vi "Test Run 1.vi"() -> ()   [LabVIEW 2009]
panel:
  out "Program Counter":u16 format="%x"
  out "Device Vcc":i32
  out "error out 2":errorcluster
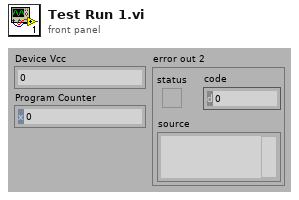
[diagram p1: front panel]
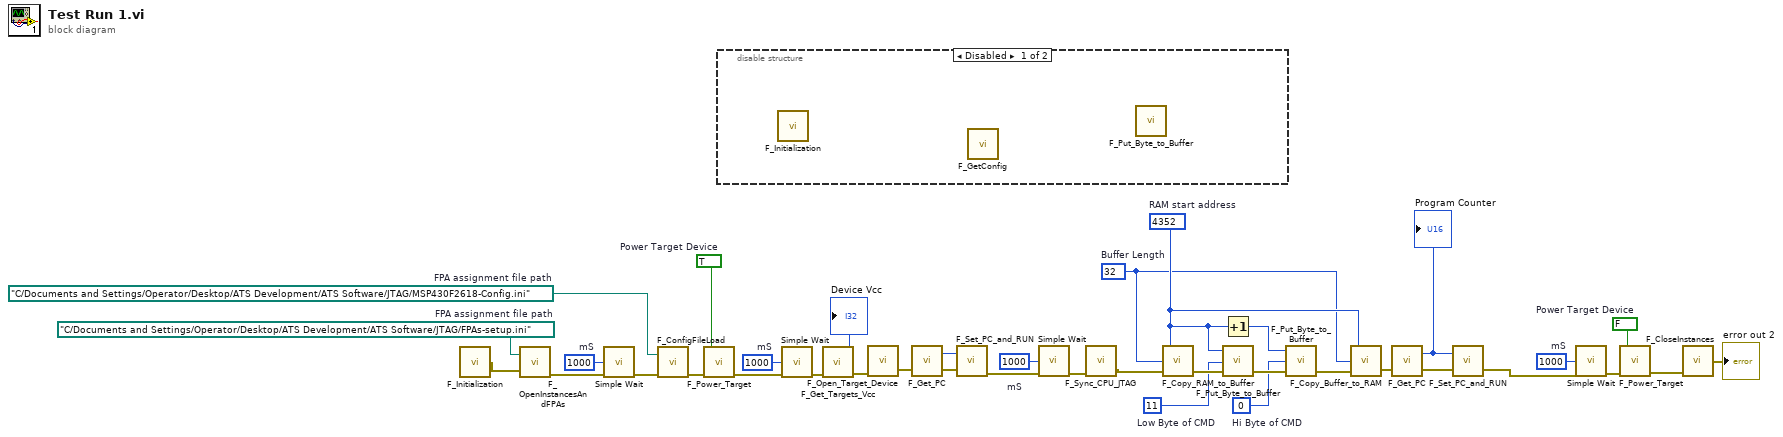
[diagram p0: block diagram]
diagram:
  w6 = u32 1000  # mS
  w15 = u32 1000  # mS
  w19 = u16 0  # Hi Byte of CMD
  w20 = u16 11  # Low Byte of CMD
  w16 = u16 32  # Buffer Length
  w17 = u16 4352  # RAM start address
  w27 = u32 1000  # mS
  w31 = FALSE  # Power Target Device
  w32 = TRUE  # Power Target Device
  w33 = path "C:/Documents and Settings/Operator/Desktop/ATS Development/ATS Software/JTAG/MSP430F2618-Config.ini"  # FPA assignment file path
  w35 = u32 1000  # mS
  w37 = path "C:/Documents and Settings/Operator/Desktop/ATS Development/ATS Software/JTAG/FPAs-setup.ini"  # FPA assignment file path
  n1 = call "F_Initialization.vi"() -> ("error out"=w1:errorcluster)  [unwired: 1 in]
  n2 = call "F_OpenInstancesAndFPAs.vi"("error in (no error)"=w1, "FPA assignment file path"=w37) -> ("error out"=w36:errorcluster)  [unwired: 1 out]
  n3 = call "Simple Wait.vi"("mS"=w35, "error in"=w36) -> ("error out"=w34:errorcluster)  [unwired: 12 in, 1 out]
  n4 = call "F_ConfigFileLoad.vi"("error in (no error)"=w34, "Config file path"=w33) -> ("error out"=w4:errorcluster)  [unwired: 1 in]
  n5 = call "F_Power_Target.vi"("error in (no error)"=w4, "Power Target Device"=w32) -> ("error out"=w25:errorcluster)  [unwired: 1 in]
  n6 = disable-structure shown="Disabled" {
    frame #0 {
      n7 = call "F_Initialization.vi"() -> ()  [unwired: 1 in, 1 out]
      n8 = call "F_GetConfig.vi"() -> ()  [unwired: 2 in, 2 out]
      n9 = call "F_Put_Byte_to_Buffer.vi"() -> ()  [unwired: 5 in, 1 out]
    }
    frame #1 {
    }
  }
  n10 = call "Simple Wait.vi"("mS"=w27, "error in"=w25) -> ("error out"=w26:errorcluster)  [unwired: 12 in, 1 out]
  n11 = call "F_Get_Targets_Vcc.vi"("error in (no error)"=w26) -> ("error out"=w24:errorcluster, "Device Vcc"=→"Device Vcc":i32)  [unwired: 1 in]
  n12 = call "F_Open_Target_Device.vi"("error in (no error)"=w24) -> ("error out"=w7:errorcluster)
  n13 = call "F_Get_PC.vi"("error in (no error)"=w7) -> ("error out"=w8:errorcluster, "Program Counter"=w9:u16)  [unwired: 1 in]
  n14 = call "F_Set_PC_and_RUN.vi"("error in (no error)"=w8, "PC start address"=w9) -> ("error out"=w5:errorcluster)  [unwired: 1 in]
  n15 = call "Simple Wait.vi"("mS"=w6, "error in"=w5) -> ("error out"=w3:errorcluster)  [unwired: 12 in, 1 out]
  n16 = call "F_Sync_CPU_JTAG.vi"("error in (no error)"=w3) -> ("error out"=w2:errorcluster)  [unwired: 1 in, 1 out]
  n17 = call "F_Copy_RAM_to_Buffer.vi"("error in (no error)"=w2, "Block size to be copied"=w16, "RAM start address"=w17) -> ("error out"=w23:errorcluster)  [unwired: 2 in]
  n18 = Increment(x=w17) -> (x+1=w21:u16)
  n19 = call "F_Put_Byte_to_Buffer.vi"("error in (no error)"=w23, "New value"=w20, "Address of byte to be updated"=w17) -> ("error out"=w22:errorcluster)  [unwired: 2 in]
  n20 = call "F_Put_Byte_to_Buffer.vi"("error in (no error)"=w22, "New value"=w19, "Address of byte to be updated"=w21) -> ("error out"=w18:errorcluster)  [unwired: 2 in]
  n21 = call "F_Copy_Buffer_to_RAM.vi"("error in (no error)"=w18, "Block size to be copied"=w16, "Buffer start address"=w17) -> ("error out"=w12:errorcluster)  [unwired: 2 in]
  n22 = call "F_Get_PC.vi"("error in (no error)"=w12) -> ("error out"=w10:errorcluster, "Program Counter"=w11:u16)  [unwired: 1 in]
  "Program Counter" <- w11
  n23 = call "F_Set_PC_and_RUN.vi"("error in (no error)"=w10, "PC start address"=w11) -> ("error out"=w13:errorcluster)  [unwired: 1 in]
  n24 = call "Simple Wait.vi"("mS"=w15, "error in"=w13) -> ("error out"=w14:errorcluster)  [unwired: 12 in, 1 out]
  n25 = call "F_Power_Target.vi"("error in (no error)"=w14, "Power Target Device"=w31) -> ("error out"=w30:errorcluster)  [unwired: 1 in]
  n26 = call "F_CloseInstances.vi"("error in (no error)"=w30) -> ("error out"=→"error out 2":errorcluster)
